vi "draw_oval.vi"() -> ()   [LabVIEW 2019]
panel:
  out "Waveform Chart 3":dbl(graph)
  out "Waveform Chart 2":dbl(graph)
  in  "stop":bool
  out "Waveform Chart":dbl(graph)
  in  "resolution":i32
  out "XY Graph":cluster{dbl[], dbl[]}(graph)
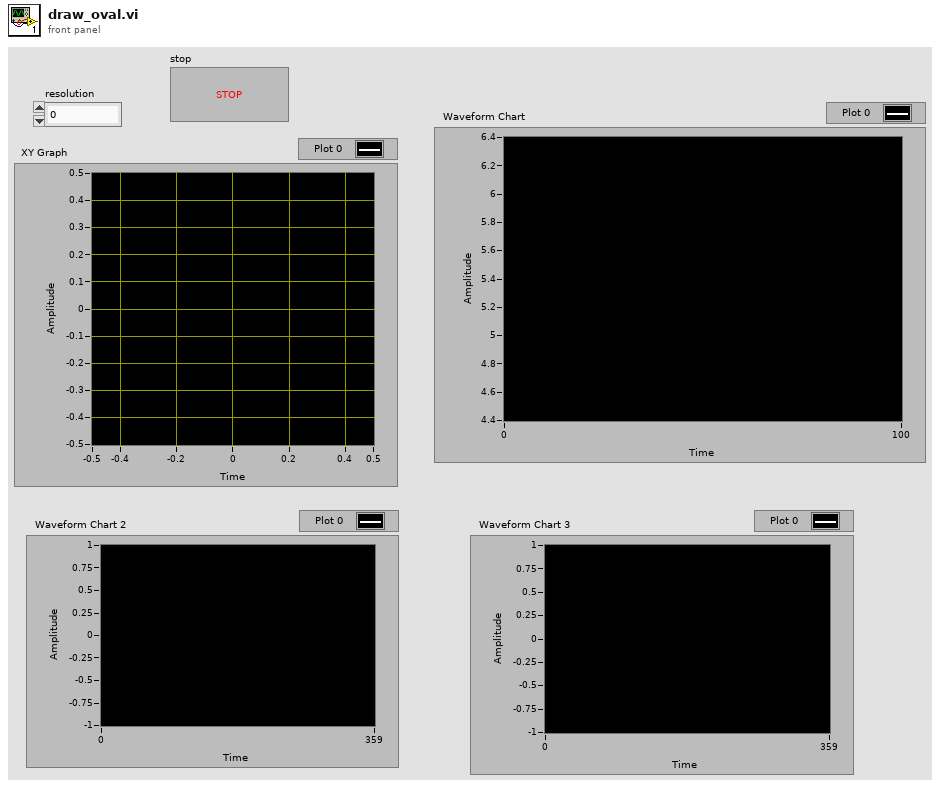
[diagram p1: front panel]
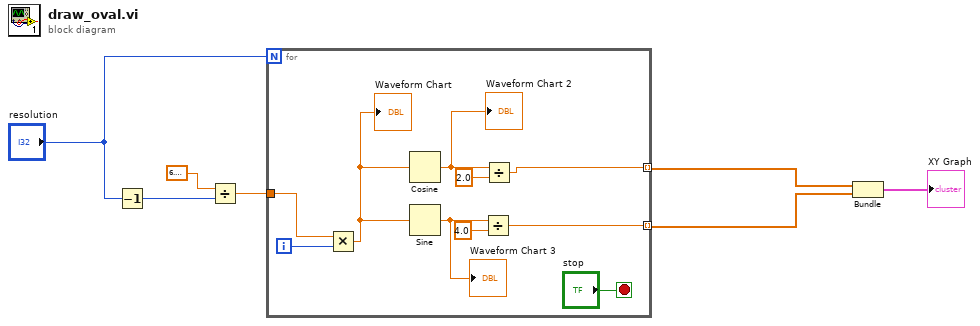
[diagram p0: block diagram]
diagram:
  n1 = Decrement(x="resolution") -> (x-1=w5:i32)
  n2 = Divide(x=6.283185307179586, y=w5) -> (x/y=w4:dbl)
  n3 = for {
    N: "resolution" -> [_]
    tunnel: w4 -> [w16]
    tunnel: [w13] -> w3 mode=indexing
    tunnel: [w14] -> w2 mode=indexing
    i -> [w17]
    stop <- "stop" stop-if-true
    n4 = Multiply(x=w16, y=w17) -> (x*y=w11:dbl)
    "Waveform Chart" <- w11
    n5 = Cosine(x=w11) -> (cos(x)=w9:dbl)
    "Waveform Chart 2" <- w9
    n6 = Sine(x=w11) -> (sin(x)=w8:dbl)
    "Waveform Chart 3" <- w8
    n7 = Divide(x=w8, y=4.0) -> (x/y=w14:dbl)
    n8 = Divide(x=w9, y=2.0) -> (x/y=w13:dbl)
  }
  n9 = Bundle(w3, w2) -> (→"XY Graph":cluster{dbl[], dbl[]})  [unwired: 1 in]
